vi "HFRR ADV v04.vi"() -> ()   [LabVIEW 2025] (continued)
                n3608 = call <vilib>:"Open_Create_Replace File.vi"("advisory dialog? (display:T)"=FALSE, "function (open:0)"=T25."create or replace", "file path"=w4584) -> ("error out"=w4597:errorcluster, "refnum"=w4596:refnum<file>)  [unwired: 5 in, 2 out]
                n3609 = Set File Position(refnum=w4596, from (0:start)=w4587, error in=w4597) -> (refnum out=w4577:refnum<file>, error out=w4576:errorcluster)  [unwired: 1 in]
                n3610 = Write to Binary File(file (use dialog)=w4577, data=" ", error in=w4576, 5:FALSE ("prepend array or string size? (T)")) -> (refnum out=w4588:refnum<file>, error out=w4589:errorcluster)  [unwired: 2 in, 1 out]
                n3611 = Set File Position(offset (in bytes) (0)=w4587, refnum=w4588, error in=w4589) -> (refnum out=w4580:refnum<file>, error out=w4579:errorcluster)  [unwired: 1 in]
                n3612 = Write to Binary File(file (use dialog)=w4580, data=w4585, error in=w4579, 5:FALSE ("prepend array or string size? (T)")) -> (error out=w4583:errorcluster)  [unwired: 2 in, 2 out]
                n3613 = flat-sequence {
                  tunnel: w4584 -> [w4599]
                  tunnel: w4583 -> [_]
                  frame #0 {
                    n3614 = call <vilib>:"Read Characters From File.vi"("file path (dialog if empty)"=w4599) -> ("character string"=→"Sensor Health JSON string":string)  [unwired: 5 in, 3 out]
                  }
                }
                "SinglePoint  2" <- w4585
              }
              frame #1 {
              }
              frame #2 {
                (unwired) "\"Stored\": true" ("string")
                n3615 = call <vilib>:"System Exec.vi"("run minimized? (F)"=TRUE, "wait until completion? (T)"=TRUE, "working directory"=path "C:/LAB-IQ-NXT", "command line"="C:\\LAB-IQ-NXT\\JPostH.bat") -> ("standard error"=→"Respose From Server 2":string, "standard output"=w4604:string)  [unwired: 4 in, 2 out]
                "standard output 2" <- w4604
                n3616 = Match Pattern(string=w4604, regular expression="JSONH Check String") -> (match substring=w4602:string, offset past match=w4601:i32)  [unwired: 1 in, 2 out]
                n3617 = Equal?(x=w4602, y="JSONH Check String") -> (x = y?=→"Upload \nConfirmed 2":bool)
              }
            }
            n3618 = Divide(x=w4444, y=3600.0 ("f")) -> (x/y=w4437:dbl)
            n3619 = local read "run time"() -> (w4494:string[])
            n3620 = Round To Nearest(number=w4437) -> (nearest integer value=w4436:dbl)
            n3621 = Number To Decimal String(number=w4436) -> (decimal integer string=w4435:string)  [unwired: 1 in]
            n3622 = Index Array(array="Sensor Information", index (col) #1=0 ("disabled index (col)"), index (col) #2=1 ("index (col)"), index (col) #3=2 ("index (col)"), index (col) #4=3 ("index (col)")) -> (element #1=→"Sensor name":string[], element #2=→"model num":string[], element #3=→"run time":string[], element #4=→"state":string[])  [unwired: 4 in]
            n3623 = Insert Into Array(array=w4494, index=1, new element #1=w4435, new element #2=w4435, new element #3=w4435, new element #4=w4435, new element #5=w4435, new element #6=w4435) -> (w4459:string[])
            "run" <- w4459
            n3624 = local read "out"() -> (w4441:string[])
            n3625 = local read "Sensor Information"() -> (w4461:string[][])
            n3626 = Replace Array Subset(array=w4461, new element #1=w4459, index (col) #1=2 ("disabled index (col)"), new element #2=w4441, index (col) #2=3 ("index (col)")) -> (w4460:string[][])  [unwired: 2 in]
            n3627 = local write "Sensor Information"(w4460) -> ()
          }
        }
        n3628 = case shown="True" w4408 {
          frame False {
          }
          frame True {
            n3629 = Equal?(x="FLAG", y=0.0) -> (x = y?=w4425:bool)
            n3630 = case shown="False" w4425 {
              frame False {
                n3631 = Get Date/Time In Seconds() -> (seconds since 1Jan1904=w4431:timestamp)
                n3632 = local read "START 2"() -> (w4429:dbl)
                n3633 = To Double Precision Float(number=w4431) -> (double precision float=w4430:dbl)
                n3634 = Subtract(x=w4430, y=w4429) -> (x-y=→"SENSOR TIME  2":dbl)
              }
              frame True {
                n3635 = Get Date/Time In Seconds() -> (seconds since 1Jan1904=w4433:timestamp)
                n3636 = To Double Precision Float(number=w4433) -> (double precision float=→"START 2":dbl)
                n3637 = local write "FLAG"(100.0 ("FLAG")) -> ()
              }
            }
          }
        }
        n3638 = disable-structure shown="Disabled" {
          disable-tunnel: w4411 -> [w4420 _]
          disable-tunnel: [w4419 _] -> w4410
          frame Disabled {
            n3639 = local read "Json St Flg"() -> (w4418:bool)
            n3640 = case shown="True" w4418 {
              tunnel: w4420 -> [w4421 w4423]
              tunnel: [w4421 w4422] -> w4419
              frame False {
              }
              frame True {
                n3641 = Increment(x=w4423) -> (x+1=w4422:dbl)
                "T cycle" <- w4422
                n3642 = local write "Json St Flg"(FALSE ("Json St Flg")) -> ()
              }
            }
          }
          frame Enabled {
          }
        }
        n3643 = local read "Quit"() -> (w4405:bool)
      }
    }
    frame Enabled {
    }
  }
  n3644 = stacked-sequence {
    tunnel: [w4803] -> w38
    frame #0 {
      w4803 = FALSE ("Upload \nConfirmed")
      n3645 = local write "Upload \nConfirmed"(w4803) -> ()
      n3646 = local write "St Str"("") -> ()
    }
  }
  n3647 = disable-structure shown="Disabled" {
    disable-tunnel: w38 -> [w4804 _]
    frame Disabled {
      n3648 = case shown="True" {
        selector: _ -> [_ _]
        tunnel: w4804 -> [_ w4805]
        frame False {
        }
        frame True {
          n3649 = while {
            tunnel: [w4811] -> _
            tunnel: w4805 -> [_]
            i -> [w4811]
            stop <- w4806 stop-if-true
            n3650 = local read "Json End Flg"() -> (w4810:bool)
            n3651 = Wait (ms)(milliseconds to wait=u32 20 ("Refresh Rate (ms)")) -> ()  [unwired: 1 out]
            n3652 = local read "refresh flag"() -> (w4807:bool)
            n3653 = local read "RUN"() -> (w4808:bool)
            n3654 = And(x=w4808, y=w4807) -> (x .and. y?=w4809:bool)
            n3655 = Or(x=w4809, y=w4810) -> (x .or. y?=w4812:bool)
            "AR Led" <- w4812
            n3656 = case shown="True" w4812 {
              frame False {
              }
              frame True {
                w4829 = "\",\""
                n3657 = local read "UUID"() -> (w4827:string)
                n3658 = local write "refresh flag"(FALSE ("refresh flag")) -> ()
                n3659 = local read "time"() -> (w4816:dbl)
                n3660 = Multiply(x=w4816, y=60.0) -> (x*y=w4815:dbl)
                n3661 = Concatenate Strings("UUID\" : \"", w4827, "\"}") -> (w4830:string)
                n3662 = Number To Fractional String(number=w4815, width (-)=i16 10, precision (6)=i16 4) -> (F-format string=w4844:string)  [unwired: 1 in]
                n3663 = Concatenate Strings("{", "\"Time\":\"", w4844, w4829) -> (w4839:string)
                n3664 = stacked-sequence {
                  tunnel: w4829 -> [w4892 w4900 w4907 w4915 w4923 w4932 w4939]
                  tunnel: [w4893 _ _ _ _ _ _] -> w4843
                  tunnel: [_ w4901 _ _ _ _ _] -> w4842
                  tunnel: [_ _ w4908 _ _ _ _] -> w4841
                  tunnel: [_ _ _ w4917 _ _ _] -> w4840
                  tunnel: w4830 -> [_ _ _ _ _ _ w4950]
                  tunnel: [_ _ _ _ _ _ w4949] -> w4826
                  tunnel: [_ _ _ _ _ w4929 _] -> w4825
                  tunnel: [_ _ _ _ w4922 _ _] -> w4824
                  frame #0 {
                    n3665 = local read "NORMAL LOAD"() -> (w4891:dbl)
                    n3666 = Number To Fractional String(number=w4891, width (-)=i16 10, precision (6)=i16 4) -> (F-format string=w4894:string)  [unwired: 1 in]
                    n3667 = Concatenate Strings("NormalLoad\":\"", w4894, w4892) -> (w4893:string)
                  }
                  frame #1 {
                    n3668 = local read "Temp"() -> (w4899:dbl)
                    n3669 = Number To Fractional String(number=w4899, width (-)=i16 10, precision (6)=i16 4) -> (F-format string=w4902:string)  [unwired: 1 in]
                    n3670 = Concatenate Strings("Temperature\":\"", w4902, w4900) -> (w4901:string)
                  }
                  frame #2 {
                    n3671 = local read "cof"() -> (w4905:dbl)
                    n3672 = Number To Fractional String(number=w4905, width (-)=i16 10, precision (6)=i16 4) -> (F-format string=w4909:string)  [unwired: 1 in]
                    n3673 = Concatenate Strings("FrictionalForce\":\"", w4909, w4907) -> (w4908:string)
                  }
                  frame #3 {
                    n3674 = local read "Set Hz"() -> (w4913:dbl)
                    n3675 = Multiply(x=w4913, y=60.0) -> (x*y=w4912:dbl)
                    n3676 = Number To Fractional String(number=w4912, width (-)=i16 10, precision (6)=i16 4) -> (F-format string=w4918:string)  [unwired: 1 in]
                    n3677 = Concatenate Strings("Speed\":\"", w4918, w4915) -> (w4917:string)
                  }
                  frame #4 {
                    n3678 = local read item#-1() -> (w4921)
                    n3679 = Number To Fractional String(number=w4921, width (-)=i16 10, precision (6)=i16 4) -> (F-format string=w4925:string)  [unwired: 1 in]
                    n3680 = Concatenate Strings("LinearDeformation\":\"", w4925, w4923) -> (w4922:string)
                  }
                  frame #5 {
                    n3681 = local read "AIR TEMP"() -> (w4928:dbl)
                    n3682 = local read "Json St Flg"() -> (w4930:bool)
                    n3683 = local read "Json End Flg"() -> (w4931:bool)
                    n3684 = Number To Fractional String(number=w4928, width (-)=i16 10, precision (6)=i16 4) -> (F-format string=w4934:string)  [unwired: 1 in]
                    n3685 = Concatenate Strings("Vibration\":\"", w4934, w4932) -> (w4929:string)
                    n3686 = And(x=w4930, y=w4931) -> ()  [unwired: 1 out]
                  }
                  frame #6 {
                    n3687 = local read "Json End Flg"() -> (w4938:bool)
                    n3688 = Get Date/Time In Seconds() -> (seconds since 1Jan1904=w4946:timestamp)
                    n3689 = local read "Json St Flg"() -> (w4937:bool)
                    n3690 = To Double Precision Float(number=w4946) -> (double precision float=w4945:dbl)
                    n3691 = Subtract(x=w4945, y=2082844800.0) -> (x-y=w4943:dbl)
                    n3692 = Number To Fractional String(number=w4943, width (-)=i16 12, precision (6)=i16 0) -> (F-format string=w4940:string)  [unwired: 1 in]
                    n3693 = case shown="True" w4938 {
                      tunnel: ["" w4953] -> w4947
                      tunnel: w4940 -> [_ w4954]
                      tunnel: w4939 -> [_ w4952]
                      frame False {
                      }
                      frame True {
                        n3694 = local write "Json End Flg"(FALSE ("Json St Flg")) -> ()
                        n3695 = Concatenate Strings("End\": \"", w4954, w4952) -> (w4953:string)
                      }
                    }
                    n3696 = case shown="True" w4937 {
                      tunnel: [w4957 w4960] -> w4948
                      tunnel: w4940 -> [_ w4961]
                      tunnel: w4939 -> [_ w4958]
                      frame False {
                        n3697 = local read "St Str"() -> (w4957:string)
                      }
                      frame True {
                        n3698 = Concatenate Strings("Start\":\"", w4961, w4958) -> (w4960:string)
                        "St Str" <- w4960
                        n3699 = local write "Json St Flg"(FALSE ("Json St Flg")) -> ()
                      }
                    }
                    n3700 = Concatenate Strings(w4948, w4947, w4950) -> (w4949:string)
                  }
                }
                n3701 = local read "FILE"() -> (w4818:string)
                n3702 = Concatenate Strings("\",\"OperatorID\":\"" ("string"), "Operator ID") -> (w4821:string)
                n3703 = Concatenate Strings("\",\"DatasetTitle\":\"" ("string"), w4818) -> (w4820:string)
                n3704 = Concatenate Strings("\",\"SerialNumber\":\"" ("string"), "Serial No") -> (w4850:string)
                n3705 = Concatenate Strings("\",\"ModelNumber\":\"" ("string"), "Model No") -> (w4849:string)
                n3706 = Concatenate Strings(w4850, w4849) -> (w4832:string)
                n3707 = Concatenate Strings("{\"SecretKey\":\"", "Secret Key", w4832, w4821, w4820, "\",\"Samples\":[") -> (w4837:string)
                n3708 = Concatenate Strings(w4839, w4843, w4842, w4841, w4840, w4824, w4825, w4826) -> (w4838:string)
                n3709 = Concatenate Strings(w4837, w4838, "]}") -> (w4836:string)
                n3710 = stacked-sequence {
                  tunnel: w4836 -> [w4865 _ _]
                  tunnel: [_ _ w4882] -> _
                  frame #0 {
                    (unwired) FALSE ("convert eol (F)")
                    w4867 = enum16{"start", "end", "current"}."start" ("pos mode (0:2)")
                    n3711 = Path To String(path="Path") -> (string=w4873:string)
                    n3712 = Concatenate Strings(w4873, "\\", "Data File Name") -> (w4875:string)
                    n3713 = local write "standard output"(" ") -> ()
                    n3714 = String To Path(string=w4875) -> (path=w4864:path)
                    n3715 = call <vilib>:"Open_Create_Replace File.vi"("advisory dialog? (display:T)"=FALSE, "function (open:0)"=T25."create or replace", "file path"=w4864) -> ("error out"=w4878:errorcluster, "refnum"=w4877:refnum<file>)  [unwired: 5 in, 2 out]
                    n3716 = Set File Position(refnum=w4877, from (0:start)=w4867, error in=w4878) -> (refnum out=w4858:refnum<file>, error out=w4857:errorcluster)  [unwired: 1 in]
                    n3717 = Write to Binary File(file (use dialog)=w4858, data=" ", error in=w4857, 5:FALSE ("prepend array or string size? (T)")) -> (refnum out=w4868:refnum<file>, error out=w4869:errorcluster)  [unwired: 2 in, 1 out]
                    n3718 = Set File Position(offset (in bytes) (0)=w4867, refnum=w4868, error in=w4869) -> (refnum out=w4861:refnum<file>, error out=w4860:errorcluster)  [unwired: 1 in]
                    n3719 = Write to Binary File(file (use dialog)=w4861, data=w4865, error in=w4860, 5:FALSE ("prepend array or string size? (T)")) -> (error out=w4863:errorcluster)  [unwired: 2 in, 2 out]
                    n3720 = flat-sequence {
                      tunnel: w4864 -> [w4880]
                      tunnel: w4863 -> [_]
                      frame #0 {
                        n3721 = call <vilib>:"Read Characters From File.vi"("file path (dialog if empty)"=w4880) -> ("character string"=→"JSON string":string)  [unwired: 5 in, 3 out]
                      }
                    }
                    "SinglePoint" <- w4865
                  }
                  frame #1 {
                  }
                  frame #2 {
                    (unwired) "\"Stored\": true" ("string")
                    n3722 = call <vilib>:"System Exec.vi"("run minimized? (F)"=TRUE, "wait until completion? (T)"=TRUE, "working directory"=path "C:/LAB-IQ-NXT", "command line"="C:\\LAB-IQ-NXT\\JPost.bat") -> ("standard error"=→"Respose From Server":string, "standard output"=w4885:string)  [unwired: 4 in, 2 out]
                    "standard output" <- w4885
                    n3723 = Match Pattern(string=w4885, regular expression="JSON Check String") -> (match substring=w4883:string, offset past match=w4882:i32)  [unwired: 1 in, 2 out]
                    n3724 = Equal?(x=w4883, y="JSON Check String") -> (x = y?=→"Upload \nConfirmed":bool)
                  }
                }
              }
            }
            n3725 = local read "Quit"() -> (w4806:bool)
          }
        }
      }
    }
    frame Enabled {
    }
  }
  n3726 = disable-structure shown="Disabled" {
    disable-tunnel: _ -> [w4968 _]
    frame Disabled {
      n3727 = while {
        shift-right: [w4976] -> w4964
        shift-left: _ -> [w4977]
        shift-right: [w4974] -> w4965
        shift-left: errorcluster {"status"=TRUE, "code"=0, "source"="Init"} ("error out") -> [w4975]
        shift-right: [w4972] -> _
        shift-left: "" -> [w4973]
        tunnel: [w4970] -> _
        tunnel: w4968 -> [_]
        i -> [w4970]
        stop <- w4969 stop-if-true
        n3728 = flat-sequence {
          tunnel: [w4978] -> w4971
          frame #0 {
            n3729 = Wait (ms)(milliseconds to wait=10.0 ("Delay")) -> (millisecond timer value=w4978:u32)
          }
        }
        n3730 = case shown="No Error" w4975 {
          selector: w4975 -> [w5008 w5127]
          tunnel: [w4991 w5129] -> w4976
          tunnel: [w4990 w5128] -> w4974
          tunnel: w4977 -> [w5009 w5121]
          tunnel: w4973 -> [w4989 w5120]
          tunnel: [w4988 w5120] -> w4972
          tunnel: w4971 -> [_ _]
          frame No Error {
            n3731 = Concatenate Strings("\r", "\n") -> (w5000:string)  [unwired: 1 in]
            n3732 = case shown="True" w5001 {
              tunnel: w5009 -> [w5033 w5040]
              tunnel: w5008 -> [w5032 w5039]
              tunnel: [w5033 w5038] -> w5007
              tunnel: [w5032 w5037] -> w4987
              tunnel: w5000 -> [_ w5036]
              frame False {
              }
              frame True {
                n3733 = VISA Write(VISA resource name=w5040, write buffer=w5036, error in (no error)=w5039) -> (VISA resource name out=w5038:refnum<visa-resource-name>, error out=w5037:errorcluster)  [unwired: 1 out]
                n3734 = local write "Read String"("") -> ()
                n3735 = local write item#-1(FALSE) -> ()
              }
            }
            n3736 = property class="Instr"(reference=w5007, error in=w4987) -> (reference out=w5006:refnum<visa-resource-name>, error out=w5005:errorcluster, "Serial Settings:Number of Bytes at Serial Port"=w5004:u32)
            n3737 = Greater?(x=w5004, y=u32 100) -> (0:w5002:bool)
            n3738 = case shown="True" w5002 {
              tunnel: w5006 -> [w5043 w5067]
              tunnel: w5005 -> [w5042 w5066]
              tunnel: w5004 -> [_ w5065]
              tunnel: [w5043 w5064] -> w4993
              tunnel: [w5042 w5063] -> w4992
              tunnel: w4989 -> [w5041 w5062]
              tunnel: [w5041 ""] -> w4988
              frame False {
              }
              frame True {
                w5052 = u32 6 ("y")
                # "Page 84 of \nmanual"
                n3739 = VISA Read(VISA resource name=w5067, byte count=w5065, error in (no error)=w5066) -> (VISA resource name out=w5064:refnum<visa-resource-name>, read buffer=w5060:string, error out=w5063:errorcluster)  [unwired: 1 out]
                n3740 = while {
                  tunnel: w5060 -> [w5116]
                  tunnel: [w5112] -> w5054 mode=indexing
                  tunnel: [w5106] -> w5058 mode=indexing
                  tunnel: [w5104] -> _
                  i -> [w5104]
                  stop <- w5109 stop-if-true
                  n3741 = String Subset(string=w5116, offset (0)=w5104) -> (substring=w5111:string)  [unwired: 1 in]
                  n3742 = String To Byte Array(string=w5111) -> (unsigned byte array=w5115:u8[])
                  n3743 = String Length(string=w5111) -> (length=w5110:i32)
                  n3744 = Index Array(array=w5115) -> (element=w5114:u8)  [unwired: 1 in]
                  n3745 = Equal To 0?(x=w5110) -> (x = 0?=w5109:bool)
                  n3746 = Number To Boolean Array(number=w5114) -> (Boolean array=w5108:bool[])
                  n3747 = Reverse 1D Array(array=w5108) -> (reversed array=w5107:bool[])
                  n3748 = And(x=w5108, y=bool[] [FALSE, FALSE, FALSE, FALSE, FALSE, FALSE, TRUE, TRUE] ("Boolean array")) -> (x .and. y?=w5112:bool[])
                  n3749 = And(x=w5107, y=bool[] [FALSE, FALSE, TRUE, TRUE, TRUE, TRUE, TRUE, TRUE] ("Boolean array")) -> (x .and. y?=w5106:bool[])
                }
                n3750 = Concatenate Strings(w5062, w5060) -> (→"Read String":string)
                n3751 = while {
                  tunnel: w5054 -> [w5103] mode=indexing
                  tunnel: [w5099] -> w5057
                  i -> [w5099]
                  stop <- w5100 stop-if-true
                  n3752 = Search 1D Array(1D array=w5103, element=TRUE) -> (index of element=w5101:i32)  [unwired: 1 in]
                  n3753 = Less Than 0?(x=w5101) -> (x < 0?=w5100:bool)
                }
                n3754 = Delete From Array(array=w5058, length=w5057, index (row)=0) -> (array with subset deleted=w5053:bool[][])  [unwired: 1 in, 1 out]
                n3755 = Array Size(array=w5053) -> (size(s)=w5055:i32[])
                n3756 = Index Array(array=w5055) -> (element=w5047:i32)  [unwired: 1 in]
                n3757 = Greater?(x=w5047, y=w5052) -> (0:w5050:bool)
                n3758 = Subtract(x=w5047, y=w5052) -> (x-y=w5051:u32)
                n3759 = Select(t=w5051, s=w5050, f=u32 0) -> (s? t:f=w5048:u32)
                n3760 = while {
                  tunnel: w5053 -> [w5086]
                  tunnel: [w5088] -> w5046 mode=indexing
                  tunnel: w5048 -> [w5070]
                  i -> [w5087]
                  stop <- w5085 stop-if-true
                  w5077 = 6 ("index")
                  w5076 = 2 ("length")
                  # "Page 65 of \nmanual"
                  n3761 = Multiply(x=u32 3 ("y"), y=w5087) -> (x*y=w5084:u32)
                  n3762 = Divide(x=u32 102 ("y"), y=u32 65520) -> (x/y=w5094:dbl)
                  n3763 = Greater Or Equal?(x=w5084, y=w5070) -> (x >= y?=w5085:bool)
                  n3764 = Index Array(array=w5086, index (row) #1=w5084) -> (element #1=w5082:bool[], element #2=w5081:bool[], element #3=w5080:bool[])  [unwired: 5 in]
                  n3765 = Reverse 1D Array(array=w5082) -> (reversed array=w5075:bool[])
                  n3766 = Reverse 1D Array(array=w5081) -> (reversed array=w5079:bool[])
                  n3767 = Reverse 1D Array(array=w5080) -> (reversed array=w5078:bool[])
                  n3768 = Delete From Array(array=w5075, length=w5076, index=w5077) -> (array with subset deleted=w5071:bool[])  [unwired: 1 out]
                  n3769 = Delete From Array(array=w5079, length=w5076, index=w5077) -> (array with subset deleted=w5072:bool[])  [unwired: 1 out]
                  n3770 = Delete From Array(array=w5078, length=w5076, index=w5077) -> (array with subset deleted=w5073:bool[])  [unwired: 1 out]
                  n3771 = Insert Into Array(array=bool[] [] ("Boolean array"), new element #1=w5071, new element #2=w5072, new element #3=w5073) -> (w5074:bool[])  [unwired: 1 in]
                  n3772 = Boolean Array To Number(Boolean array=w5074) -> (number=w5083:u32)
                  n3773 = Multiply(x=w5094, y=w5083) -> (x*y=w5093:dbl)
                  n3774 = Decrement(x=w5093) -> (x-1=w5092:dbl)
                  n3775 = Divide(x=w5092, y=u32 100) -> (x/y=w5090:dbl)
                  n3776 = Multiply(x=w5090, y=u32 10) -> (x*y=w5088:dbl)
                }
                n3777 = Delete From Array(array=w5046) -> (array with subset deleted=w5045:dbl[])  [unwired: 2 in, 1 out]
                "Waveform Graph 5" <- w5045
                "Waveform Chart 3" <- w5045
                n3778 = call-poly <vilib>:"Mean.vi"("X"=w5045) -> ("mean"=w5044:dbl)  [unwired: 1 out]
                n3779 = case shown="True" {
                  selector: _ -> [_ _]
                  tunnel: w5044 -> [_ w5069]
                  frame False {
                  }
                  frame True {
                    n3780 = local write item#-1(FALSE ("Zero 4")) -> ()
                    "z_measure" <- w5069
                  }
                }
              }
            }
            n3781 = local read item#-1() -> (w4984)
            n3782 = local read item#-1() -> (w4983)
            n3783 = local read item#-1() -> (w4985)
            n3784 = local read item#-1() -> (w4982)
            n3785 = case shown="True" w4980 {
              tunnel: w4984 -> [_ w5012]
              tunnel: w4985 -> [_ w5011]
              frame False {
              }
              frame True {
                n3786 = Build Array(w5012, w5011) -> (w5010:void[])
                n3787 = local read item#-1() -> (w5015)
                n3788 = Build Array (concatenate)(w5015, w5010) -> (w5013:void[])
                n3789 = local write item#-1(w5013) -> ()
                n3790 = local write item#-1(FALSE ("Boolean 8")) -> ()
              }
            }
            n3791 = call "Build XY Graph"("Enable"=w4982, "Reset"=w4983, "Y Input"=w4985, "X Input"=w4984) -> ("XY Graph"=w4981:cluster{"Y":dbl[], "Y":dbl[]}[])  [unwired: 6 in, 1 out]
            n3792 = case shown="True" {
              selector: _ -> [_ _]
              frame False {
              }
              frame True {
                n3793 = local read item#-1() -> (w5016)
                n3794 = Index Array(array=w5016, index (col) #1=0 ("disabled index (col)"), index (col) #2=1 ("index (col)")) -> (element #1=w5018, element #2=w5017)  [unwired: 2 in]
                n3795 = call <vilib>:"Linear Fit.vi"("Y"=w5018, "X"=w5017) -> ()  [unwired: 9 in, 5 out]
                n3796 = local write item#-1(FALSE ("Boolean 9")) -> ()
              }
            }
            n3797 = case shown="True" {
              selector: _ -> [_ _]
              frame False {
              }
              frame True {
                n3798 = local write item#-1(dbl[][] [] ("Captured Values")) -> ()
                n3799 = local write item#-1(FALSE ("Boolean 7")) -> ()
              }
            }
            n3800 = Concatenate Strings("\r", "\n") -> (w4995:string, w4994:string)
            n3801 = case shown="True" w4986 {
              tunnel: w4993 -> [w5025 w5031]
              tunnel: w4992 -> [w5024 w5030]
              tunnel: [w5025 w5029] -> w4991
              tunnel: [w5024 w5028] -> w4990
              tunnel: w4995 -> [_ w5027]
              frame False {
              }
              frame True {
                n3802 = VISA Write(VISA resource name=w5031, write buffer=w5027, error in (no error)=w5030) -> (VISA resource name out=w5029:refnum<visa-resource-name>, error out=w5028:errorcluster)  [unwired: 1 out]
                n3803 = local write item#-1(FALSE ("WRITE")) -> ()
              }
            }
          }
          frame Error {
            w5119 = u16 10 items=["1.0"=10, "1.5"=15, "2.0"=20] ("stop bits (10: 1 bit)")
            n3804 = Wait (ms)(milliseconds to wait=u32 20) -> ()  [unwired: 1 out]
            n3805 = VISA Close(VISA resource name=w5121, error in (no error)=w5127) -> (error out=w5126:errorcluster)
            n3806 = call <vilib>:"Clear Errors.vi"("error in (no error)"=w5126) -> ("error out"=w5125:errorcluster)  [unwired: 5 in, 1 out]
            n3807 = call-poly "VISA Configure Serial Port"("timeout (10sec)"=u32 200, "Enable Termination\nChar (T)"=TRUE ("Enable Termination\nChar (T)"), "baud rate (9600)"=u32 921600, "error in (no error)"=w5125, "stop bits (10: 1 bit)"=w5119) -> ("VISA resource name"=w5117:refnum<visa-resource-name>, "VISA resource name out"=w5129:refnum<visa-resource-name>, "error out"=w5128:errorcluster)  [unwired: 8 in]
          }
        }
        n3808 = local read "Quit"() -> (w4969:bool)
      }
      n3809 = VISA Close(VISA resource name=w4964, error in (no error)=w4965) -> (error out=w4963:errorcluster)
      n3810 = call <vilib>:"Clear Errors.vi"("error in (no error)"=w4963) -> ()  [unwired: 5 in, 2 out]
    }
    frame Enabled {
    }
  }
  n3811 = disable-structure shown="Disabled" {
    disable-tunnel: _ -> [w5134 _]
    frame Disabled {
      n3812 = while {
        tunnel: [w5141] -> _
        shift-right: [w5138] -> w5131
        shift-left: _ -> [w5140]
        shift-right: [w5139] -> w5132
        shift-left: errorcluster {"status"=TRUE, "code"=0, "source"="Init"} ("error out") -> [w5137]
        tunnel: w5134 -> [_]
        i -> [w5141]
        stop <- w5135 stop-if-true
        n3813 = flat-sequence {
          tunnel: w5137 -> [w5232]
          tunnel: [w5232] -> w5136
          frame #0 {
            n3814 = Wait (ms)(milliseconds to wait=u32 50) -> ()  [unwired: 1 out]
          }
        }
        n3815 = case shown="No Error" w5136 {
          selector: w5136 -> [w5182 w5225]
          tunnel: w5140 -> [w5181 w5224]
          tunnel: [w5148 w5215] -> w5139
          tunnel: [w5149 w5223] -> w5138
          frame No Error {
            w5175 = T26 {"Mode"=enum."RTU", "Slave Address"=1} ("Serial Parameters")
            n3816 = call-poly <vilib>:"MB Serial Master Query (poly).vi"("VISA resource name"=w5181, "Starting Address"=i16 1000, "Quantity"=u16 1, "Timeout"=u32 1000, "error in"=w5182, "Serial Parameters"=w5175) -> ("VISA resource name out"=w5176:refnum<visa-resource-name>, "Input Registers"=w5178:u16[], "error out"=w5174:errorcluster)  [unwired: 10 in, 1 out]
            n3817 = Random Number (0-1)() -> (number: 0 to 1=w5163:dbl)
            n3818 = Index Array(array=w5178, index=0) -> (element=w5173:u16)
            n3819 = Subtract(x=w5163, y=0.5) -> (x-y=w5162:dbl)
            n3820 = Divide(x=w5173, y=10 ("index")) -> (x/y=w5167:dbl)
            n3821 = Multiply(x=w5162, y=0.5) -> (x*y=w5161:dbl)
            n3822 = Add(x=w5167, y=w5161) -> (x+y=w5166:dbl)
            n3823 = local read "Amb temp"() -> (w5150:dbl)
            n3824 = Multiply(x=w5166, y=0.2) -> (x*y=w5170:dbl)
            n3825 = Multiply(x=w5150, y=0.8) -> (x*y=w5168:dbl)
            n3826 = Add(x=w5170, y=w5168) -> (x+y=w5151:dbl)
            n3827 = local read "set temp old"() -> (w5145:dbl)
            n3828 = local write "Amb temp"(w5151) -> ()
            n3829 = Select(t="SetTemp 2", s="Heater", f=100.0) -> (s? t:f=w5146:dbl)
            n3830 = Not Equal?(x=w5146, y=w5145) -> (x != y?=w5144:bool)
            n3831 = case shown="True" w5144 {
              tunnel: w5176 -> [w5210 w5212]
              tunnel: [w5209 w5212] -> w5156
              tunnel: w5174 -> [w5208 w5211]
              tunnel: [w5207 w5211] -> w5154
              tunnel: w5146 -> [w5202 _]
              tunnel: w5175 -> [w5204 w5213]
              tunnel: [w5204 w5213] -> w5157
              frame True {
                n3832 = Multiply(x=w5202, y=10 ("index")) -> (x*y=w5201:dbl)
                n3833 = call-poly <vilib>:"MB Serial Master Query (poly).vi"("VISA resource name"=w5210, "Address"=u16 0, "Holding Register"=w5201, "Timeout"=u32 1000, "error in"=w5208, "Serial Parameters"=w5204) -> ("VISA resource name out"=w5209:refnum<visa-resource-name>, "error out"=w5207:errorcluster)  [unwired: 11 in, 1 out]
                "set temp old" <- w5202
              }
              frame False {
              }
            }
            n3834 = flat-sequence {
              tunnel: [w5183] -> _
              tunnel: [w5183] -> w5153
              tunnel: w5154 -> [w5183]
              frame #0 {
                n3835 = Wait (ms)(milliseconds to wait=u32 100) -> ()  [unwired: 1 out]
              }
            }
            n3836 = call "Elapsed Time12"("Time Target (s)"=2.0, "Auto Reset"=TRUE) -> ("Time has Elapsed"=w5158:bool)  [unwired: 10 in, 7 out]
            n3837 = case shown="True" w5158 {
              tunnel: w5157 -> [w5187 w5200]
              tunnel: [w5187 w5200] -> _
              tunnel: [w5186 w5198] -> w5149
              tunnel: w5156 -> [w5186 w5199]
              tunnel: [w5185 w5196] -> w5148
              tunnel: w5153 -> [w5185 w5197]
              frame False {
              }
              frame True {
                n3838 = call-poly <vilib>:"MB Serial Master Query (poly).vi"("VISA resource name"=w5199, "Starting Address"=i16 1003 ("Addr"), "Quantity"=u16 1, "Timeout"=u32 1000, "error in"=w5197, "Serial Parameters"=w5200) -> ("VISA resource name out"=w5198:refnum<visa-resource-name>, "Input Registers"=w5193:u16[], "error out"=w5196:errorcluster)  [unwired: 10 in, 1 out]
                n3839 = Index Array(array=w5193, index=0) -> (element=w5192:u16)
                n3840 = Divide(x=w5192, y=u16 10) -> (x/y=w5188:dbl)
                n3841 = local write "set temp old"(w5188) -> ()
                n3842 = local write "SetTemp"(w5188) -> ()
              }
            }
            "Error Code" <- w5148
            n3843 = Unbundle(w5148) -> ("status"=→"TK4 status":bool)  [unwired: 2 out]
            "SetTemp" <- "SetTemp 2"
          }
          frame Error {
            w5227 = u16 0 items=["None", "Odd", "Even", "Mark", "Space"] ("Parity")
            w5228 = u16 0 items=["None", "XON/XOFF", "RTS/CTS", "XON/XOFF & RTS/CTS", "DTR/DSR", "XON/XOFF & DTR/DSR"] ("Flow Control")
            n3844 = VISA Clear(VISA resource name=w5224, error in (no error)=w5225) -> (VISA resource name out=w5218:refnum<visa-resource-name>, error out=w5216:errorcluster)
            n3845 = VISA Close(VISA resource name=w5218, error in (no error)=w5216) -> (error out=w5217:errorcluster)
            n3846 = call <vilib>:"Clear Errors.vi"("error in (no error)"=w5217) -> ("error out"=w5226:errorcluster)  [unwired: 5 in, 1 out]
            n3847 = Unbundle By Name(T26 {"Mode"=enum."RTU", "Slave Address"=1} ("input cluster")) -> ("Mode"=w5229:enum16{"RTU", "ASCII"})
            n3848 = call <vilib>:"MB Serial Init.vi"("Timeout"=u32 100, "Flow Control"=w5228, "Mode"=w5229, "error in (no error)"=w5226, "Parity"=w5227, "Baud Rate"=u32 9600, "VISA resource name"="Lubrication System COM Port :") -> ("error out"=w5215:errorcluster, "VISA resource name out"=w5223:refnum<visa-resource-name>)  [unwired: 3 in]
            n3849 = local write "set temp old"(0.0 ("set temp old")) -> ()
            n3850 = Unbundle(w5215) -> ("status"=w5214:bool)  [unwired: 2 out]
            n3851 = case shown="True" w5214 {
              selector: w5214 -> [_ w5231]
              frame False {
              }
              frame True {
                n3852 = local write "TK4 status"(w5231) -> ()
              }
            }
          }
        }
        n3853 = local read "Quit"() -> (w5135:bool)
      }
      n3854 = VISA Close(VISA resource name=w5131, error in (no error)=w5132) -> (error out=w5130:errorcluster)
      n3855 = call <vilib>:"Clear Errors.vi"("error in (no error)"=w5130) -> ()  [unwired: 5 in, 2 out]
    }
    frame Enabled {
    }
  }
